vi "Create Number of Tags.vi"(0 "NumberOfTags":i32, 11 "error in (no error)":errorcluster) -> (4 "TagsArray":refnum<class "Tag.lvclass">[](array[class]), 15 "error out":errorcluster)   [LabVIEW 2014, in "Tag.lvclass"]
doc: "This VI creates x number of tags."
uses:
  Tag.lvclass
  Global FieldLengthX.vi
  Global FieldWidthY.vi
panel:
  out "error out 2":errorcluster caption="error out"
  in  "error in (no error) 2":errorcluster caption="error in (no error)"
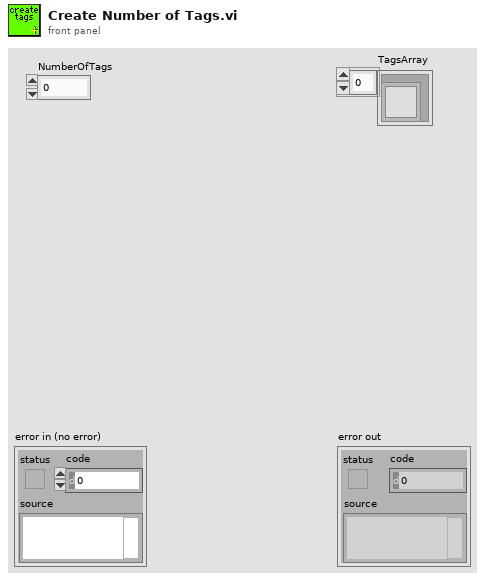
[diagram p1: front panel]
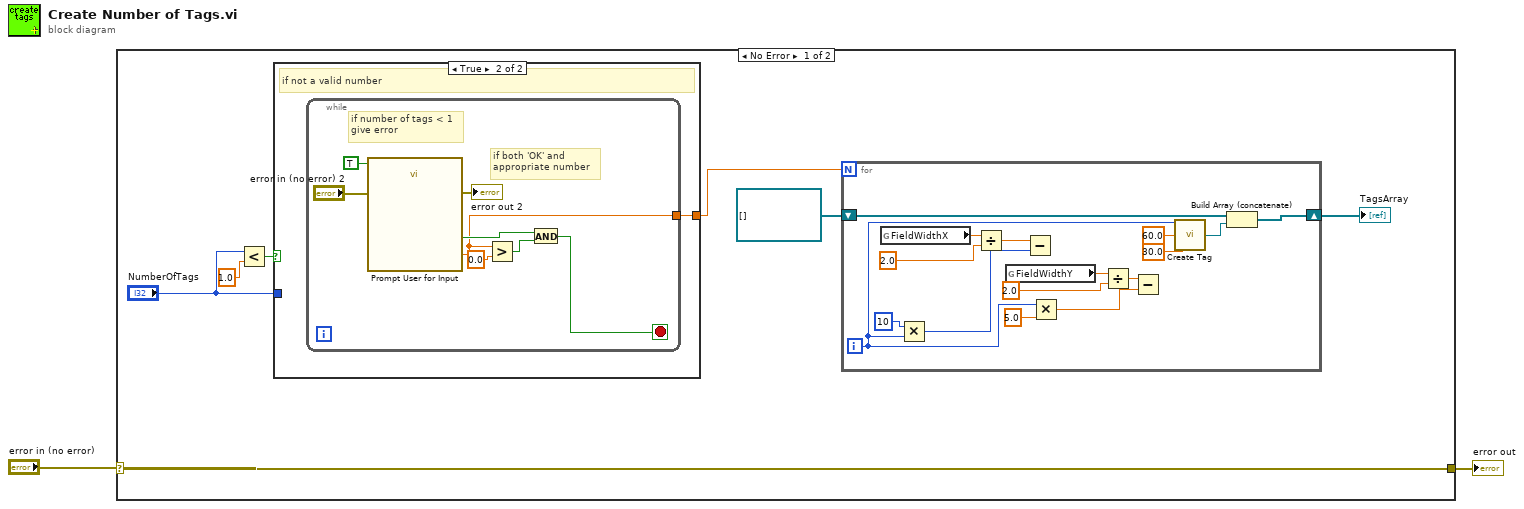
[diagram p0: block diagram]
diagram:
  n1 = case shown="No Error" "error in (no error)" {
    selector: "error in (no error)" -> [w9 w36]
    tunnel: [w9 w36] -> w1
    frame No Error {
      n2 = Less?(x="NumberOfTags", y=1.0) -> (x < y?=w6:bool)
      n3 = case shown="True" w6 {
        tunnel: "NumberOfTags" -> [w10 _]
        tunnel: [w10 w11] -> w8
        frame False {
        }
        frame True {
          # "if not a valid number"
          n4 = while {
            tunnel: [w13] -> w11
            stop <- w12 stop-if-true
            # "if both 'OK' and \nappropriate number"
            # "if number of tags < 1\ngive error"
            n5 = call "Prompt User for Input"("Enable"=TRUE, "error in (no error)"="error in (no error) 2") -> ("number"=w13:dbl, "OK"=w14:bool, "error out"=→"error out 2":errorcluster)  [unwired: 15 in]
            n6 = Greater?(x=w13, y=0.0) -> (0:w15:bool)
            n7 = And(x=w14, y=w15) -> (x .and. y?=w12:bool)
          }
        }
      }
      n8 = for {
        N: w8 -> [_]
        shift-right: [w23] -> w4
        shift-left: refnum<class "Tag.lvclass">[] [] -> [w25]
        i -> [w22]
        n9 = global read "Global FieldLengthX.vi" "FieldWidthX"() -> (w34:dbl)
        n10 = Multiply(x=10, y=w22) -> (x*y=w27:i32)
        n11 = Divide(x=w34, y=2.0) -> (x/y=w35:dbl)
        n12 = global read "Global FieldWidthY.vi" "FieldWidthY"() -> (w32:dbl)
        n13 = Subtract(x=w35, y=w27) -> ()  [unwired: 1 out]
        n14 = Multiply(x=w22, y=5.0) -> (x*y=w26:dbl)
        n15 = Divide(x=w32, y=2.0) -> (x/y=w30:dbl)
        n16 = Subtract(x=w30, y=w26) -> ()  [unwired: 1 out]
        n17 = call "Create Tag.vi"("TagY"=30.0, "TagX"=60.0, "TagID"=w22) -> ("Tag Out"=w24:refnum<class "Tag.lvclass">)
        n18 = Build Array (concatenate)(w25, w24) -> (w23:refnum<class "Tag.lvclass">[])
      }
      "TagsArray" <- w4
    }
    frame Error {
    }
  }
  "error out" <- w1
